vi "Agilent PSG MXG_IDN.vi"(11 "IDN String":string) -> ()   [LabVIEW 2015]
uses:
  <vilib>/regexp/Match Regular Expression.xnode
panel:
  out "Match?":bool
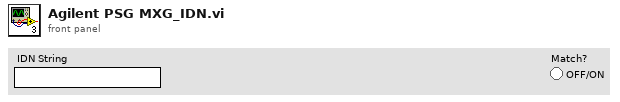
[diagram p1: front panel]
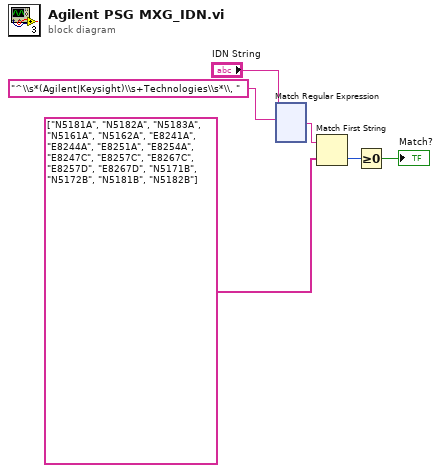
[diagram p0: block diagram]
diagram:
  n1 = xnode ("Match Regular Expression")("input string"="IDN String", "regular expression"="^\\s*(Agilent|Keysight)\\s+Technologies\\s*\\, " ("Company Name Regular Expression")) -> ("after match"=w4:string)  [unwired: 4 in, 4 out]
  n2 = Match First String(2:string[] ["N5181A", "N5182A", "N5183A", "N5161A", "N5162A", "E8241A", "E8244A", "E8251A", "E8254A", "E8247C", "E8257C", "E8267C", "E8257D", "E8267D", "N5171B", "N5172B", "N5181B", "N5182B"], 3:w4) -> (0:w2:i32)  [unwired: 1 out]
  n3 = Greater Or Equal To 0?(x=w2) -> (x >= 0?=→"Match?":bool)
